vi "Untitled 1.vi"() -> ()   [LabVIEW 2014]
panel:
  out "test":bool
  in  "test":bool
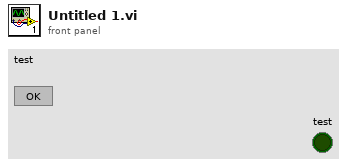
[diagram p1: front panel]
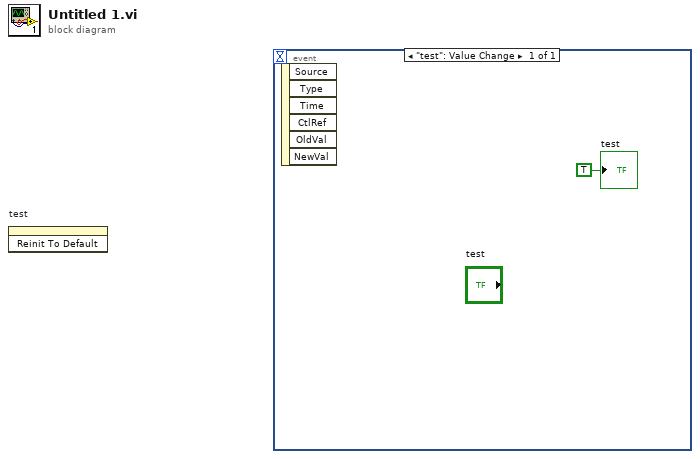
[diagram p0: block diagram]
diagram:
  n1 = invoke on="test" class="Bool" method="Reinit To Default"() -> ()  [unwired: 3 in, 3 out]
  n2 = event shown="[0] \"test\": Value Change" {
    selector: _ -> [_]
    dyn-events: _ -> [_]
    timeout: _ -> [_]
    event "test": Value Change {
      n3 = event-data() -> ()  [unwired: 1 in, 6 out]
      "test" <- TRUE ("test")
    }
  }
